vi "Write data Stop Bit.vi"(9 "stop bit":bool, 11 "WT1600.lvlib:1600Card.lvlib:1600 Card Actor.lvclass":refnum<class "1600 Card Actor.lvclass">) -> (3 "1600 Card Actor out":refnum<class "1600 Card Actor.lvclass">)   [LabVIEW 2012, in "WT1600.lvlib" / "1600Card.lvlib" / "1600 Card Actor.lvclass"]
uses:
  1600 Card Actor.lvclass
  1600 Card Actor.lvclass/1600 Card Actor.ctl
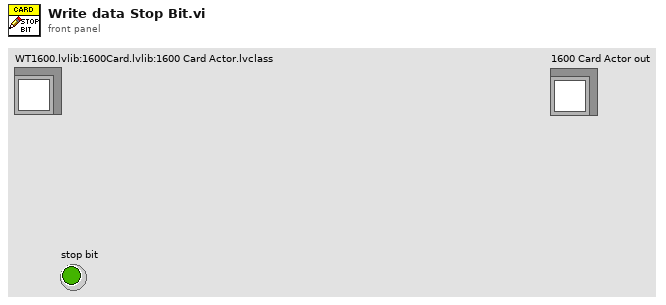
[diagram p1: front panel]
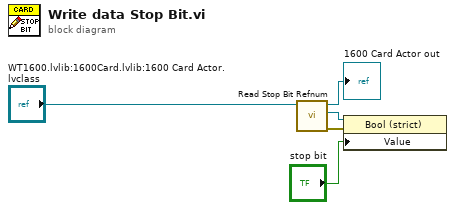
[diagram p0: block diagram]
diagram:
  n1 = call "Read Stop Bit Refnum.vi"("1600 Card Actor in"="WT1600.lvlib:1600Card.lvlib:1600 Card Actor.lvclass") -> ("error out"=w2:errorcluster, "Stop Bit Refnum"=w3:refnum<vi>, "1600 Card Actor out"=→"1600 Card Actor out":refnum<class "1600 Card Actor.lvclass">)  [unwired: 8 in]
  n2 = property class="Bool (strict)"(reference=w3, error in=w2, "Value"="stop bit") -> ()  [unwired: 2 out]
